vi "cRIO Personality.vi"() -> ()   [LabVIEW 2019]
uses:
  <vilib>/NI/NI VeriStand Development Tools/NI Veristand FPGA Specialty IO/Types/QuadratureEncoder.Measure.Digital.Settings.ctl
  <vilib>/NI/NI VeriStand Development Tools/NI Veristand FPGA Specialty IO/Types/QuadratureEncoder.Measure.Digital.Measurement.ctl
  <vilib>/NI/NI VeriStand Development Tools/NI Veristand FPGA Specialty IO/Types/WSS.Generate.Digital.Settings.ctl
  <vilib>/NI/NI VeriStand Development Tools/NI Veristand FPGA Specialty IO/Types/Static.Measure.Digital.Measurement.ctl
  <vilib>/NI/NI VeriStand Development Tools/NI Veristand FPGA Specialty IO/Types/Static.Measure.Digital.Settings.ctl
  <vilib>/NI/NI VeriStand Development Tools/NI Veristand FPGA Specialty IO/Types/Static.Generate.Digital.Settings.ctl
  <vilib>/NI/NI VeriStand Development Tools/NI Veristand FPGA Specialty IO/Types/PWM.Generate.Digital.Settings.ctl
  <vilib>/NI/NI VeriStand Development Tools/NI Veristand FPGA Specialty IO/Types/PWM.Measure.Digital.Settings.ctl
  <vilib>/NI/NI VeriStand Development Tools/NI Veristand FPGA Specialty IO/Types/PWM.Measure.Digital.Measurement.ctl
  <vilib>/rvi/Emulation/niFpgaGetClockAttributes.vi
  <vilib>/rvi/Emulation/niFpgaSctlEmulationGetInTimedLoop.vi
  <vilib>/rvi/Emulation/niFpgaEmulationReportErrorSimple.vi
  <vilib>/rvi/Emulation/niFpgaCriticalErrorInLSC.vi
  <vilib>/NI/NI VeriStand Development Tools/NI Veristand FPGA Specialty IO/Speciality FPGA IO.lvlib
panel:
  in  "I16":i16
  in  "I8":i8
  in  "I64":i64
  in  "I32":i32
  in  "U16":u16
  in  "U8":u8
  in  "U64":u64
  in  "U32":u32
  in  "SGL":sgl
  in  "Boolean":bool
  out "I16 out":i16
  out "I8 out":i8
  out "I64 out":i64
  out "I32 out":i32
  out "U16 out":u16
  out "U8 out":u8
  out "U64 out":u64
  out "U32 out":u32
  out "SGL out":sgl
  out "Boolean out":bool
  in  "FXP24.5":fxp<+/-,24,5>
  in  "FXP16.5":fxp<+/-,16,5>
  in  "FXP32.8":fxp<+/-,32,8>
  in  "FXP64.32":fxp<+/-,64,32>
  out "FXP24.5 out":fxp<+/-,24,5>
  out "FXP16.5 out":fxp<+/-,16,5>
  out "FXP32.8 out":fxp<+/-,32,8>
  out "FXP64.32 out":fxp<+/-,64,32>
  in  "FXP16.7":fxp<+/-,16,7>
  out "FXP16.7 out":fxp<+/-,16,7>
  in  "FXP20.5":fxp<+/-,20,5>
  out "FXP20.5 out":fxp<+/-,20,5>
  in  "FXP27.5":fxp<+/-,27,5>
  out "FXP27.5 out":fxp<+/-,27,5>
  in  "FXP32.16":fxp<+/-,32,16>
  out "FXP32.16 out":fxp<+/-,32,16>
  in  "FXP16.3":fxp<+,16,3>
  out "FXP16.3 out":fxp<+,16,3>
  in  "FXP18.3":fxp<+,18,3>
  out "FXP18.3 out":fxp<+,18,3>
  in  "Group1.I16":i16
  in  "Group1.I8":i8
  in  "Group1.I64":i64
  in  "Group1.I32":i32
  in  "Group1.U16":u16
  in  "Group1.U8":u8
  in  "Group1.U64":u64
  in  "Group1.U32":u32
  in  "Group1.SGL":sgl
  in  "Group1.Boolean":bool
  out "Group1.I16 out":i16
  out "Group1.I8 out":i8
  out "Group1.I64 out":i64
  out "Group1.I32 out":i32
  out "Group1.U16 out":u16
  out "Group1.U8 out":u8
  out "Group1.U64 out":u64
  out "Group1.U32 out":u32
  out "Group1.SGL out":sgl
  out "Group1.Boolean out":bool
  in  "Group1.FXP24.5":fxp<+/-,24,5>
  in  "Group1.FXP16.5":fxp<+/-,16,5>
  in  "Group1.FXP32.8":fxp<+/-,32,8>
  in  "Group1.FXP64.32":fxp<+/-,64,32>
  out "Group1.FXP24.5 out":fxp<+/-,24,5>
  out "Group1.FXP16.5 out":fxp<+/-,16,5>
  out "Group1.FXP32.8 out":fxp<+/-,32,8>
  out "Group1.FXP64.32 out":fxp<+/-,64,32>
  in  "Group1.FXP16.7":fxp<+/-,16,7>
  out "Group1.FXP16.7 out":fxp<+/-,16,7>
  in  "Group1.FXP20.5":fxp<+/-,20,5>
  out "Group1.FXP20.5 out":fxp<+/-,20,5>
  in  "Group1.FXP27.5":fxp<+/-,27,5>
  out "Group1.FXP27.5 out":fxp<+/-,27,5>
  in  "Group1.FXP32.16":fxp<+/-,32,16>
  out "Group1.FXP32.16 out":fxp<+/-,32,16>
  in  "Group1.FXP16.3":fxp<+,16,3>
  out "Group1.FXP16.3 out":fxp<+,16,3>
  in  "Group1.FXP18.3":fxp<+,18,3>
  out "Group1.FXP18.3 out":fxp<+,18,3>
  out "Measure.Digital.Ch0":T1={"ACTIVE TICKS"=4000, "INACTIVE TICKS"=12000, "ACQ TICKS"=1}
  out "Measure.Digital.Ch1":T1
  in  "Measure.Digital.Ch0.Settings":T2={"ACTIVE EDGE"=TRUE, "TIMEOUT"=40000000}
  in  "Measure.Digital.Ch1.Settings":T2={"ACTIVE EDGE"=FALSE, "TIMEOUT"=40000000}
  in  "Generate.Digital.Ch0.Internal.Settings":T3={"ACTIVE EDGE"=TRUE, "ACTIVE TICKS"=4000, "INACTIVE TICKS"=12000}
  in  "Generate.Digital.Ch1.Internal.Settings":T3={"ACTIVE EDGE"=FALSE, "ACTIVE TICKS"=60000000, "INACTIVE TICKS"=20000000}
  in  "Generate.Digital.Ch2.Internal.Settings":T4={"ACTIVE EDGE"=TRUE, "OUTPUT"=FALSE}
  in  "Measure.Digital.Ch2.Internal.Settings":T5={"ACTIVE EDGE"=TRUE}
  out "Measure.Digital.Ch2":T6
  in  "Generate.Digital.Ch3.Internal.Settings":T4={"ACTIVE EDGE"=TRUE, "OUTPUT"=FALSE}
  in  "Measure.Digital.Ch3.Internal.Settings":T5={"ACTIVE EDGE"=TRUE}
  out "Measure.Digital.Ch3":T6
  in  "Generate.Digital.Ch4.WSS.Settings":T7={"ACTIVE EDGE"=TRUE, "ACTIVE TICKS"=0, "INACTIVE TICKS"=0, "DATA"=0, "SENSOR TYPE"=0}
  out "Bit0":bool
  out "Bit1":bool
  out "Measurement.Digital.Ch5":T8
  in  "A":bool
  in  "B":bool
  in  "Z":bool
  in  "Measure.Digital.Ch5.QuadEncoder.Settings":T9={"DIRECTION"=0, "RESET VALUE"=0, "A RESET STATE"=TRUE, "B RESET STATE"=TRUE, "Z RESET STATE"=TRUE}
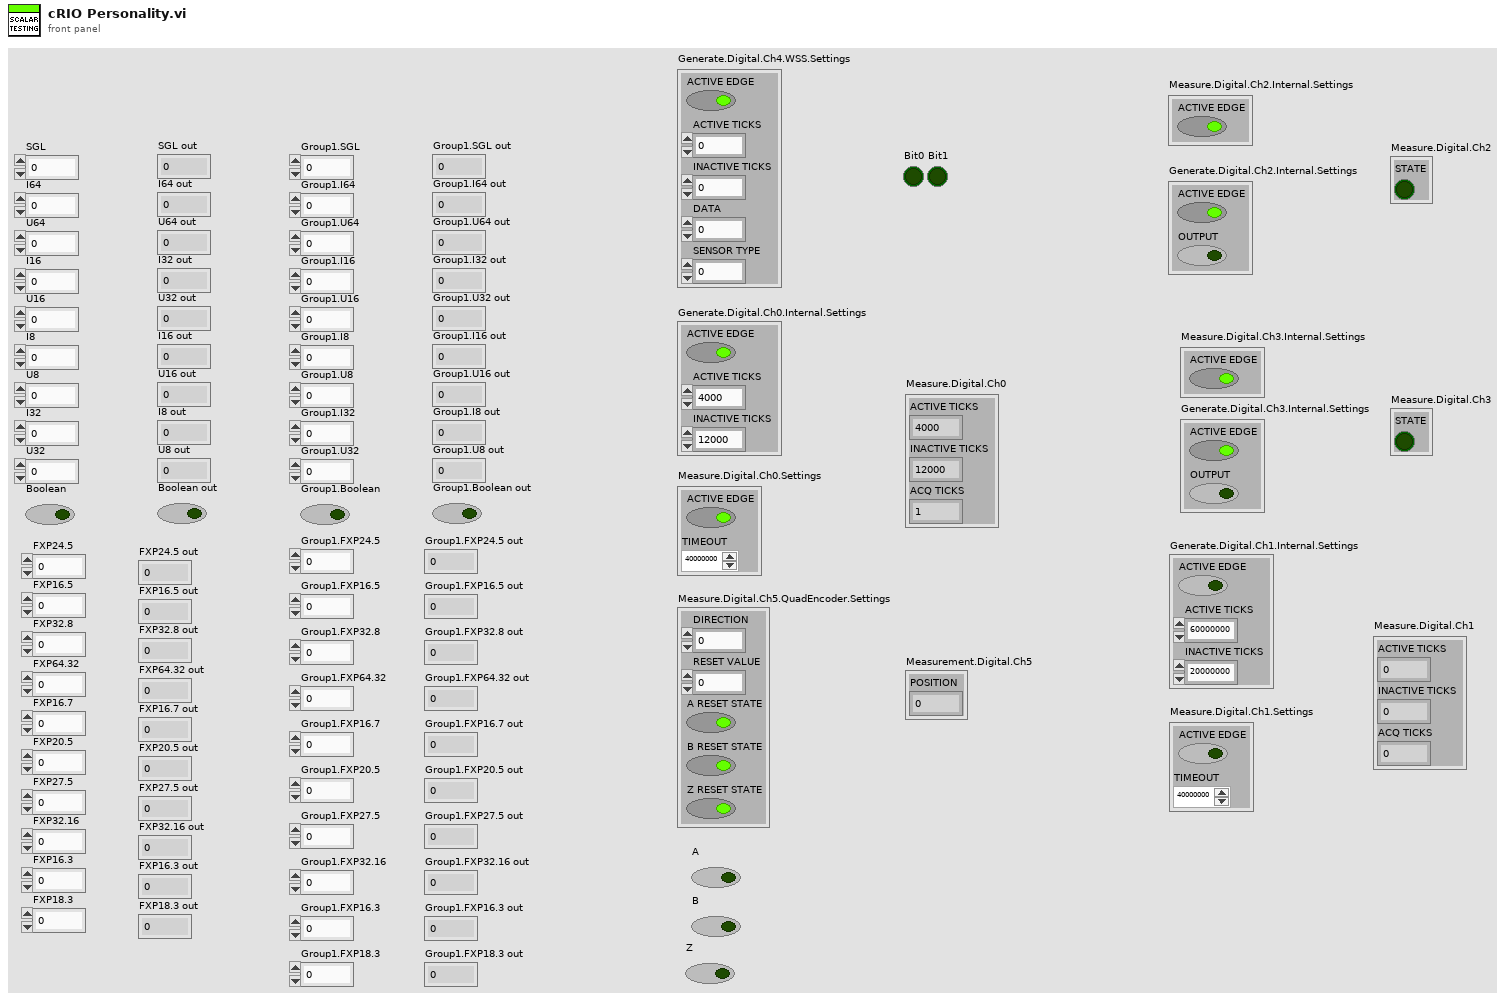
[diagram p1: front panel]
types:
  T1 = typedef "Speciality FPGA IO.lvlib/PWM.Measure.Digital.Measurement.ctl" = cluster{"ACTIVE TICKS":u32, "INACTIVE TICKS":u32, "ACQ TICKS":u32}
  T2 = typedef "Speciality FPGA IO.lvlib/PWM.Measure.Digital.Settings.ctl" = cluster{"ACTIVE EDGE":bool, "TIMEOUT":u32}
  T3 = typedef "Speciality FPGA IO.lvlib/PWM.Generate.Digital.Settings.ctl" = cluster{"ACTIVE EDGE":bool, "ACTIVE TICKS":u32, "INACTIVE TICKS":u32}
  T4 = typedef "Speciality FPGA IO.lvlib/Static.Generate.Digital.Settings.ctl" = cluster{"ACTIVE EDGE":bool, "OUTPUT":bool}
  T5 = typedef "Speciality FPGA IO.lvlib/Static.Measure.Digital.Settings.ctl" = cluster{"ACTIVE EDGE":bool}
  T6 = typedef "Speciality FPGA IO.lvlib/Static.Measure.Digital.Measurement.ctl" = cluster{"STATE":bool}
  T7 = typedef "Speciality FPGA IO.lvlib/WSS.Generate.Digital.Settings.ctl" = cluster{"ACTIVE EDGE":bool, "ACTIVE TICKS":u32, "INACTIVE TICKS":u32, "DATA":u8, "SENSOR TYPE":u8}
  T8 = typedef "Speciality FPGA IO.lvlib/QuadratureEncoder.Measure.Digital.Measurement.ctl" = cluster{"POSITION":i32}
  T9 = typedef "Speciality FPGA IO.lvlib/QuadratureEncoder.Measure.Digital.Settings.ctl" = cluster{"DIRECTION":u8, "RESET VALUE":i32, "A RESET STATE":bool, "B RESET STATE":bool, "Z RESET STATE":bool}
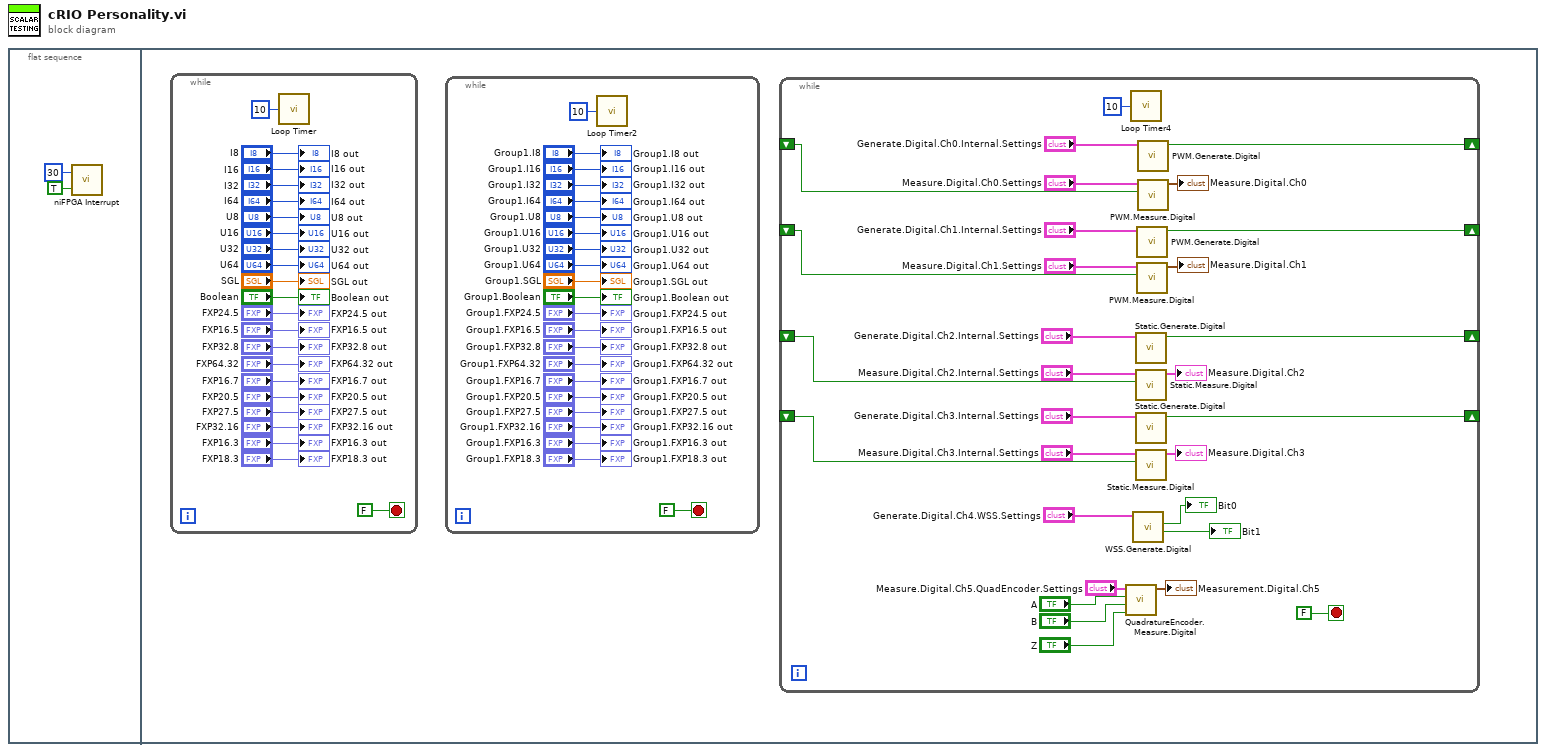
[diagram p0: block diagram]
diagram:
  n1 = flat-sequence {
    frame #0 {
      n2 = call <vilib>:"niFPGA Interrupt.vi"("Wait Until Cleared (F)"=TRUE, "IRQ Number (0)"=u8 30) -> ()  [unwired: 1 in]
    }
    frame #1 {
      n3 = while {
        stop <- FALSE stop-if-true
        n4 = call "Loop Timer"("Count(uSec)"=u32 10) -> ()  [unwired: 1 out]
        "I16 out" <- "I16"
        "I8 out" <- "I8"
        "I64 out" <- "I64"
        "I32 out" <- "I32"
        "U16 out" <- "U16"
        "U8 out" <- "U8"
        "U64 out" <- "U64"
        "U32 out" <- "U32"
        "SGL out" <- "SGL"
        "Boolean out" <- "Boolean"
        "FXP24.5 out" <- "FXP24.5"
        "FXP16.5 out" <- "FXP16.5"
        "FXP32.8 out" <- "FXP32.8"
        "FXP64.32 out" <- "FXP64.32"
        "FXP16.7 out" <- "FXP16.7"
        "FXP20.5 out" <- "FXP20.5"
        "FXP27.5 out" <- "FXP27.5"
        "FXP32.16 out" <- "FXP32.16"
        "FXP16.3 out" <- "FXP16.3"
        "FXP18.3 out" <- "FXP18.3"
      }
      n5 = while {
        stop <- FALSE stop-if-true
        n6 = call "Loop Timer2"("Count(uSec)"=u32 10) -> ()  [unwired: 1 out]
        "Group1.I16 out" <- "Group1.I16"
        "Group1.I8 out" <- "Group1.I8"
        "Group1.I64 out" <- "Group1.I64"
        "Group1.I32 out" <- "Group1.I32"
        "Group1.U16 out" <- "Group1.U16"
        "Group1.U8 out" <- "Group1.U8"
        "Group1.U64 out" <- "Group1.U64"
        "Group1.U32 out" <- "Group1.U32"
        "Group1.SGL out" <- "Group1.SGL"
        "Group1.Boolean out" <- "Group1.Boolean"
        "Group1.FXP24.5 out" <- "Group1.FXP24.5"
        "Group1.FXP16.5 out" <- "Group1.FXP16.5"
        "Group1.FXP32.8 out" <- "Group1.FXP32.8"
        "Group1.FXP64.32 out" <- "Group1.FXP64.32"
        "Group1.FXP16.7 out" <- "Group1.FXP16.7"
        "Group1.FXP20.5 out" <- "Group1.FXP20.5"
        "Group1.FXP27.5 out" <- "Group1.FXP27.5"
        "Group1.FXP32.16 out" <- "Group1.FXP32.16"
        "Group1.FXP16.3 out" <- "Group1.FXP16.3"
        "Group1.FXP18.3 out" <- "Group1.FXP18.3"
      }
      n7 = while {
        shift-right: [w31] -> _
        shift-left: _ -> [w30]
        shift-right: [w29] -> _
        shift-left: _ -> [w28]
        shift-right: [w21] -> _
        shift-left: _ -> [w19]
        shift-right: [w12] -> _
        shift-left: _ -> [w14]
        stop <- FALSE stop-if-true
        n8 = call <vilib>:"QuadratureEncoder.Measure.Digital.vi"("Z"="Z", "B"="B", "A"="A", "Settings"="Measure.Digital.Ch5.QuadEncoder.Settings") -> ("Measurement"=→"Measurement.Digital.Ch5":T8)  [unwired: 7 in]
        n9 = call "Loop Timer4"("Count(uSec)"=u32 10) -> ()  [unwired: 1 out]
        n10 = call <vilib>:"WSS.Generate.Digital.vi"("Settings"="Generate.Digital.Ch4.WSS.Settings") -> ("Bit1"=→"Bit1":bool, "Bit0"=→"Bit0":bool)  [unwired: 8 in, 1 out]
        n11 = call <vilib>:"Static.Generate.Digital.vi"("Settings"="Generate.Digital.Ch2.Internal.Settings") -> ("Output"=w21:bool)  [unwired: 10 in]
        n12 = call <vilib>:"Static.Measure.Digital.vi"("State"=w19, "Settings"="Measure.Digital.Ch2.Internal.Settings") -> ("Measurement"=→"Measure.Digital.Ch2":T6)  [unwired: 9 in]
        n13 = call <vilib>:"Static.Generate.Digital.vi"("Settings"="Generate.Digital.Ch3.Internal.Settings") -> ("Output"=w12:bool)  [unwired: 10 in]
        n14 = call <vilib>:"Static.Measure.Digital.vi"("State"=w14, "Settings"="Measure.Digital.Ch3.Internal.Settings") -> ("Measurement"=→"Measure.Digital.Ch3":T6)  [unwired: 9 in]
        n15 = call <vilib>:"PWM.Generate.Digital.vi"("Settings"="Generate.Digital.Ch1.Internal.Settings") -> ("Output"=w31:bool)  [unwired: 10 in]
        n16 = call <vilib>:"PWM.Measure.Digital.vi"("State"=w30, "Settings"="Measure.Digital.Ch1.Settings") -> ("Measurement"=→"Measure.Digital.Ch1":T1)  [unwired: 8 in, 1 out]
        n17 = call <vilib>:"PWM.Generate.Digital.vi"("Settings"="Generate.Digital.Ch0.Internal.Settings") -> ("Output"=w29:bool)  [unwired: 10 in]
        n18 = call <vilib>:"PWM.Measure.Digital.vi"("State"=w28, "Settings"="Measure.Digital.Ch0.Settings") -> ("Measurement"=→"Measure.Digital.Ch0":T1)  [unwired: 8 in, 1 out]
      }
    }
  }
